vi "solar_cfg Write (Var).vi"(0 "Config Refnum":refnum<data-value>, 1 "Section":string, 2 "Comments (Key,Comment)":cluster{"Key":string, "Comment":string}[](array[cluster]), 5 "Key (\"\")":string, 7 "Variant":variant, 9 "Include Variant Name? (F)":bool, 11 "error in (no error)":errorcluster, 12 "ArrayDelimiters (1D,2D)":string[](array[string])) -> (4 "dup Config Refnum":refnum<data-value>, 10 "Found?":bool, 15 "error out":errorcluster)   [LabVIEW 2018]
doc: "Write the values associated with a variant to a specified section in the configuration file. If the Key is empty the variant label is used instead. Set a Comment (#...) to add a description after the key's value. Clusters use the element lables are their key names. Set Enum as Strings to True to use the string item of an enum.\n\nSupported Data Types: \nI8..EXT, Enum, Boolean, String, Path, VISA Reference, Timestamp\n1D & 2D Arrays and Clusters of the data types above.\n\n[Section]\nKey = \"Value\" #Comment"
uses:
  <vilib>/Utility/Data Type/NI_Data Type.lvlib
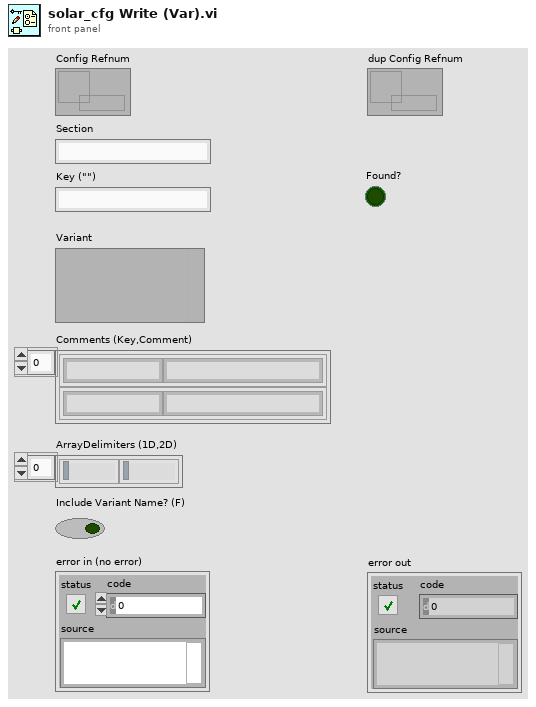
[diagram p1: front panel]
types:
  T1 = typedef "NI_Data Type.lvlib/Data Type.ctl" = enum8{"Invalid Type", "Void", "I8", "I16", "I32", "I64", "U8", "U16", "U32", "U64", "Single Float", "Double Float", "Extended Float", "Single Complex", "Double Complex", "Extended Complex", "Enum U8", "Enum U16", "Enum U32", "Enum U64", "Single Float With Unit", "Double Float With Unit", "Extended Float With Unit", "Single Complex with Unit", "Double Complex with Unit", "Extended Complex with Unit", "Boolean", "String", "Path", "Picture", "Tag", "Array", "Cluster", "Variant", "LV Variant", "Waveform", "Timestamp", "Digital Waveform", "Digital Data", "ExpressData", "Refnum", "External Data", "VI", "Poly VI", "LabVIEW Class Instance", "Fixed Point", "Set Collection", "Map Collection"}
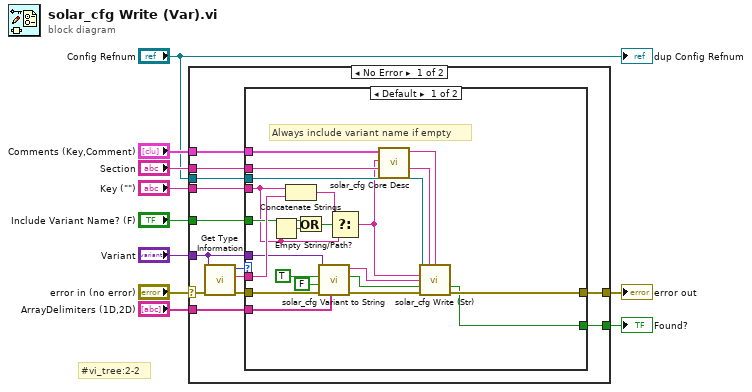
[diagram p0: block diagram]
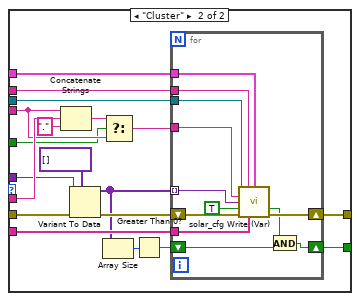
[diagram p2: hidden frame]
diagram:
  # "#vi_tree:2-2"
  n1 = case shown="No Error" "error in (no error)" {
    selector: "error in (no error)" -> [w16 w76]
    tunnel: [w22 w76] -> w9
    tunnel: "Variant" -> [w12 _]
    tunnel: "Config Refnum" -> [w20 _]
    tunnel: "Comments (Key,Comment)" -> [w23 _]
    tunnel: "Section" -> [w21 _]
    tunnel: "Key (\"\")" -> [w18 _]
    tunnel: "ArrayDelimiters (1D,2D)" -> [w17 _]
    tunnel: [w19 _] -> w6
    tunnel: "Include Variant Name? (F)" -> [w11 _]
    frame No Error {
      n2 = call <vilib>:"Get Type Information.vi"("error in (no error)"=w16, "variant"=w12) -> ("error out"=w15:errorcluster, "name"=w13:string, "type"=w14:T1)  [unwired: 5 in, 2 out]
      n3 = case shown="Default" w14 {
        tunnel: w23 -> [w42 w63]
        tunnel: [w31 w62] -> w22
        tunnel: w21 -> [w40 w61]
        tunnel: w20 -> [w43 w60]
        tunnel: [w30 w59] -> w19
        tunnel: w18 -> [w24 w50]
        tunnel: w17 -> [w32 w56]
        tunnel: w15 -> [w39 w52]
        tunnel: w13 -> [w41 w51]
        tunnel: w12 -> [w37 w49]
        tunnel: w11 -> [w25 w45]
        frame Default {
          # "Always include variant name if empty"
          n4 = Empty String/Path?(string/path=w24) -> (empty?=w29:bool)
          n5 = Concatenate Strings(w24, w41) -> (w27:string)
          n6 = Or(x=w25, y=w29) -> (x .or. y?=w28:bool)
          n7 = call "solar_cfg Variant to String.vi"("ArrayDelimiters (1D,2D)"=w32, "error in (no error)"=w39, "Boolean as 0,1? (F)"=FALSE, "Use Enum Names? (F)"=TRUE, "Variant"=w37) -> ("error out"=w38:errorcluster, "Quotes Recommended?"=w35:bool, "String"=w36:string)  [unwired: 3 in, 1 out]
          n8 = Select(t=w27, s=w28, f=w24) -> (s? t:f=w26:string)
          n9 = call "solar_cfg Core Desc.vi"("Key"=w26, "Comments (Key,Comment)"=w42) -> ("Comment"=w44:string)  [unwired: 9 in]
          n10 = call "solar_cfg Write (Str).vi"("Config Refnum"=w43, "Section"=w40, "Comment"=w44, "Key"=w26, "Value in"=w36, "Add Quotes? (T)"=w35, "error in (no error)"=w38) -> ("Found?"=w30:bool, "error out"=w31:errorcluster)  [unwired: 6 in, 1 out]
        }
        frame "Cluster" {
          n11 = Concatenate Strings(w50, w51, "." ("string")) -> (w53:string)
          n12 = Variant To Data(error in=w52, type=variant[] [], Variant=w49) -> (data=w47:variant[], error out=w48:errorcluster)
          n13 = Array Size(array=w47) -> (size(s)=w58:i32)
          n14 = Select(t=w53, s=w45, f=w50) -> (s? t:f=w46:string)
          n15 = Greater Than 0?(x=w58) -> (x > 0?=w57:bool)
          n16 = for {
            tunnel: w61 -> [w70]
            shift-right: [w67] -> w62
            shift-left: w48 -> [w73]
            tunnel: w47 -> [w72] mode=indexing
            tunnel: w63 -> [w69]
            shift-right: [w74] -> w59
            shift-left: w57 -> [w75]
            tunnel: w60 -> [w68]
            tunnel: w56 -> [w65]
            tunnel: w46 -> [w71]
            n17 = call "solar_cfg Write (Var).vi"("Config Refnum"=w68, "Section"=w70, "Comments (Key,Comment)"=w69, "Key (\"\")"=w71, "Variant"=w72, "Include Variant Name? (F)"=TRUE ("Include Cluster Name? (T)"), "error in (no error)"=w73, "ArrayDelimiters (1D,2D)"=w65) -> ("Found?"=w66:bool, "error out"=w67:errorcluster)  [unwired: 5 in, 1 out]
            n18 = And(x=w66, y=w75) -> (x .and. y?=w74:bool)
          }
        }
      }
    }
    frame Error {
    }
  }
  "error out" <- w9
  "Found?" <- w6
  "dup Config Refnum" <- "Config Refnum"
